vi "RxCALOFF.vi"(11 "VISA resource name":string) -> ()   [LabVIEW 2015]
uses:
  VISAOperation.ctl
  ONOFF.ctl
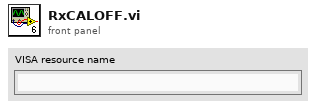
[diagram p1: front panel]
types:
  T1 = typedef "ONOFF.ctl" = u16
  T2 = typedef "VISAOperation.ctl" = enum16{"RunFile", "OpenDebugPanel", "ReadError", "ReadSTB", "Reset", "Clean", "CloseVISA", "RunCMD", "OpenVISA"}
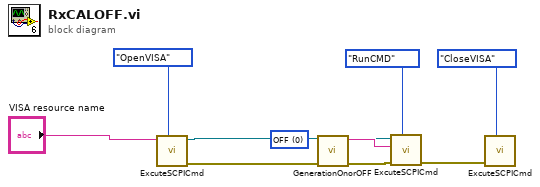
[diagram p0: block diagram]
diagram:
  w2 = T1 0 items=["OFF", "ON"] ("ON/OFF")
  n1 = call "ExcuteSCPICmd.vi"("VISAOperation"=VISAOperation."OpenVISA", "VISA resource name"="VISA resource name") -> ("error out"=w3:errorcluster, "reference out"=w4:refnum<visa-resource-name>)  [unwired: 6 in, 2 out]
  n2 = call "GenerationOnorOFF.vi"("error in (no error)"=w3, "ON/OFF"=w2) -> ("error out"=w6:errorcluster, "ON/OFFCMD"=w8:string)  [unwired: 8 in]
  n3 = call "ExcuteSCPICmd.vi"("VISAOperation"=VISAOperation."RunCMD", "error in (no error)"=w6, "Run Command"=w8, "VISA resource name"=w4) -> ("error out"=w5:errorcluster)  [unwired: 4 in, 3 out]
  n4 = call "ExcuteSCPICmd.vi"("VISAOperation"=VISAOperation."CloseVISA", "error in (no error)"=w5) -> ()  [unwired: 6 in, 4 out]
